vi "Enumerator go Next.vi"(8 "error in (no error)":errorcluster, 11 "List in":refnum<class "DoublyLinkedList.lvclass">) -> (0 "error out":errorcluster, 3 "List out":refnum<class "DoublyLinkedList.lvclass">)   [LabVIEW 2021, in "DoublyLinkedList.lvclass"]
uses:
  DoublyLinkedList.lvclass
  DoublyLinkedList.lvclass/DoublyLinkedList.ctl
  IDoublyNode/IDoublyNode.lvclass
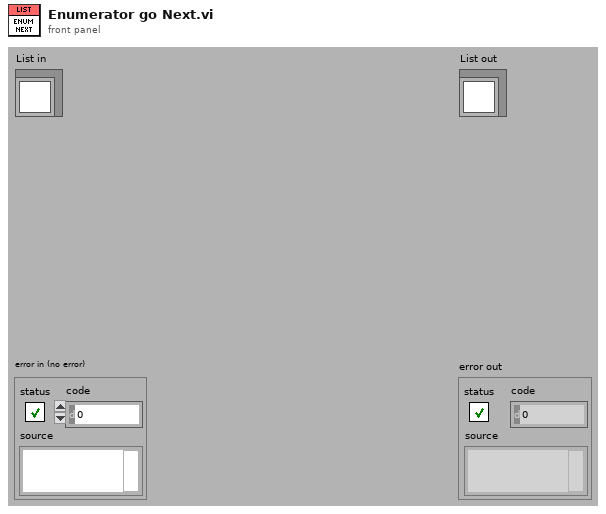
[diagram p1: front panel]
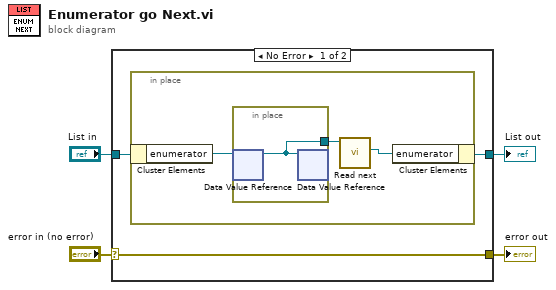
[diagram p0: block diagram]
diagram:
  n1 = case shown="No Error" "error in (no error)" {
    selector: "error in (no error)" -> [w7 w13]
    tunnel: [w7 w13] -> w3
    tunnel: [w5 w12] -> w1
    tunnel: "List in" -> [w6 w12]
    frame No Error {
      n2 = in-place {
        n3 = in-place-cluster #1(w6) -> ("enumerator"=w9:refnum<data-value>)
        n4 = in-place {
          in-place-border: [w11] -> w8
          n5 = in-place-dvr #2(w9) -> (w11:refnum<class "IDoublyNode.lvclass">)  [unwired: 1 out]
          n6 = in-place-dvr #2(w11) -> ()  [unwired: 2 out]
        }
        n7 = call-dynamic "Read next.vi"("NodeType in"=w8) -> ("next"=w10:refnum<data-value>)  [unwired: 8 in, 2 out]
        n8 = in-place-cluster #1("enumerator"=w10) -> (w5:refnum<class "DoublyLinkedList.lvclass">)
      }
    }
    frame Error {
    }
  }
  "error out" <- w3
  "List out" <- w1
